vi "MT Generate ASK system parameters (M).vi"(0 "samples per symbol (16)":i32=16, 5 "M-ASK (2)":i32=2, 11 "error in (no error)":errorcluster) -> (6 "ASK system parameters":T1 {"symbol map" format="%.3f"}, 8 "bits per symbol":i32, 15 "error out":errorcluster)   [LabVIEW 2020, in "niDMT.lvlib"]
doc: "This polymorphic instance calculates parameters for use with either the MT Modulate ASK VI or the MT Demodulate ASK VI. It accepts an M-ary value that specifies a predefined symbol map with the number of distinct levels to use as symbols."
uses:
  <vilib>/addons/Modulation/niDMT.lvlib
  <vilib>/addons/Modulation/Digital/Support/Controls/ASK system parameters.ctl
  <vilib>/addons/Modulation/niAMT.lvlib
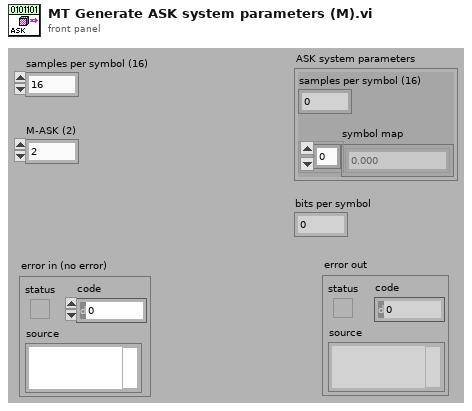
[diagram p1: front panel]
types:
  T1 = cluster{"samples per symbol (16)":i32, "symbol map":cdb[]}
  T2 = typedef "niDMT.lvlib/ASK system parameters.ctl" = cluster{"samples per symbol (16)":i32, "symbol map":cdb[]}
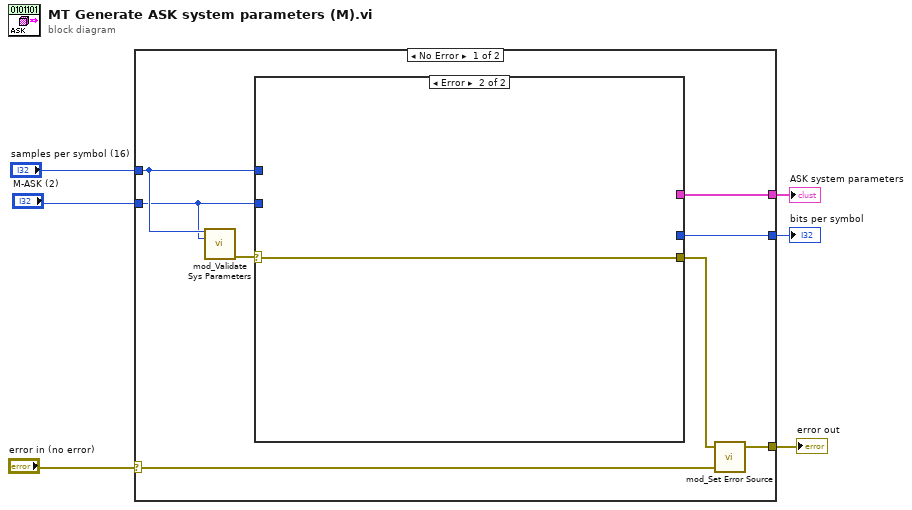
[diagram p0: block diagram]
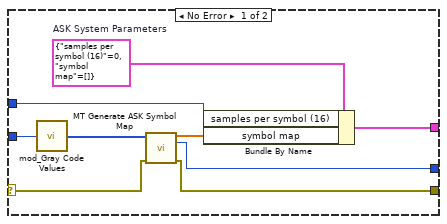
[diagram p2: hidden frame]
diagram:
  n1 = case shown="No Error" "error in (no error)" {
    selector: "error in (no error)" -> [w12 w25]
    tunnel: "M-ASK (2)" -> [w7 _]
    tunnel: [w14 _] -> w5
    tunnel: [w13 _] -> w4
    tunnel: [w11 w25] -> w3
    tunnel: "samples per symbol (16)" -> [w8 _]
    frame No Error {
      n2 = call <vilib>:"mod_Validate Sys Parameters.vi"("samples per symbol"=w8, "M-ary"=w7) -> ("error out"=w9:errorcluster)  [unwired: 13 out]
      n3 = case shown="Error" w9 {
        selector: w9 -> [w16 w24]
        tunnel: w7 -> [w23 _]
        tunnel: w8 -> [w20 _]
        tunnel: [w19 _] -> w14
        tunnel: [w18 _] -> w13
        tunnel: [w17 w24] -> w10
        frame No Error {
          w15 = T2 {"samples per symbol (16)"=0, "symbol map"=[]}  # ASK System Parameters
          n4 = call <vilib>:"mod_Gray Code Values.vi"("M"=w23) -> ("Gray coded values"=w22:i32[])
          n5 = call <vilib>:"MT Generate ASK Symbol Map.vi"("symbol values"=w22, "error in (no error)"=w16) -> ("symbol map"=w21:cdb[], "bits per symbol"=w18:i32, "error out"=w17:errorcluster)  [unwired: 11 out]
          n6 = Bundle By Name(cluster=w15, "samples per symbol (16)"=w20, "symbol map"=w21) -> (w19:T2)
        }
        frame Error {
        }
      }
      n7 = call <vilib>:"mod_Set Error Source.vi"("initial error in (no error)"=w12, "final error in (no error)"=w10) -> ("error out"=w11:errorcluster)  [unwired: 3 out]
    }
    frame Error {
    }
  }
  "ASK system parameters" <- w5
  "bits per symbol" <- w4
  "error out" <- w3
